vi "Read Configuration.vi"(8 "error in (no error)":errorcluster, 11 "Common Measurements in":refnum<class "Common Measurements.lvclass">) -> (0 "error out":errorcluster, 3 "Common Measurements out":refnum<class "Common Measurements.lvclass">)   [LabVIEW 2015, in "Common Measurements.lvclass"]
uses:
  Common Measurements.lvclass
  <vilib>/Utility/sysdir.llb/System Directory Type.ctl
  Common Measurements.lvclass/Common Measurements.ctl
  <vilib>/Utility/config.llb/Read Key (Boolean).vi
  <vilib>/Utility/config.llb/NI_LVConfig.lvlib
panel:
  out "system directory":path
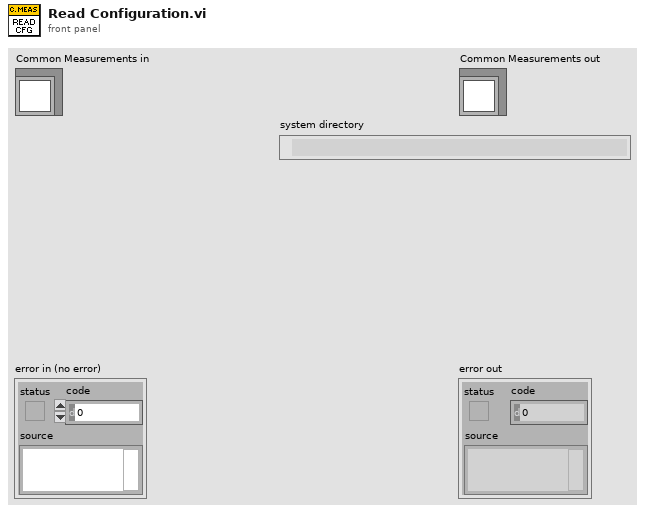
[diagram p1: front panel]
types:
  T1 = typedef "System Directory Type.ctl" = i32
  T2 = typedef "NI_LVConfig.lvlib/Config Data RefNum.ctl" = refnum<k1>
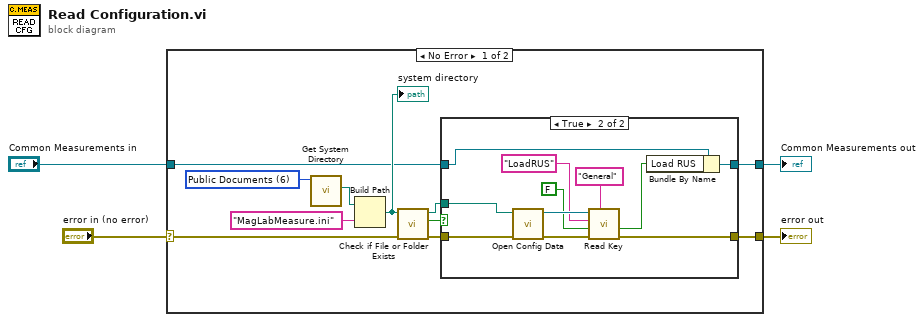
[diagram p0: block diagram]
diagram:
  n1 = case shown="No Error" "error in (no error)" {
    selector: "error in (no error)" -> [w6 w30]
    tunnel: [w5 w30] -> w3
    tunnel: [w8 w29] -> w1
    tunnel: "Common Measurements in" -> [w9 w29]
    frame No Error {
      w15 = T1 6 items=["User Home"=0, "User Desktop"=1, "User Documents"=2, "User Application Data"=3, "User Preferences"=4, "User Temporary"=5, "Public Documents"=6, "Public Application Data"=7, "Public Preferences"=8, "Public Cache"=13, "System Core Libraries"=9, "System Installed Libraries"=10, "Application Files"=11, "Boot Volume Root"=12] ("system directory type")
      n2 = call <vilib>:"Get System Directory.vi"("system directory type"=w15) -> ("system directory"=w14:path)  [unwired: 10 in]
      n3 = Build Path(base path=w14, name or relative path="MagLabMeasure.ini") -> (appended path=w12:path)
      "system directory" <- w12
      n4 = call <vilib>:"Check if File or Folder Exists.vi"("error in (no error)"=w6, "path"=w12) -> ("error out"=w7:errorcluster, "file or folder exists?"=w11:bool, "dup path"=w10:path)  [unwired: 7 in]
      n5 = case shown="True" w11 {
        tunnel: w10 -> [_ w28]
        tunnel: w9 -> [w17 w23]
        tunnel: [w17 w21] -> w8
        tunnel: w7 -> [w16 w20]
        tunnel: [w16 w19] -> w5
        frame False {
        }
        frame True {
          n6 = call <vilib>:"Open Config Data.vi"("error in (no error)"=w20, "configuration file path"=w28) -> ("error out"=w27:errorcluster, "refnum"=w26:T2)  [unwired: 7 in, 1 out]
          n7 = call-poly <vilib>:"Read Key.vi"("section"="General", "error in (no error)"=w27, "default value"=FALSE, "key"="LoadRUS", "refnum"=w26) -> ("error out"=w19:errorcluster, "value"=w22:bool)  [unwired: 3 in, 2 out]
          n8 = Bundle By Name(cluster=w23, "Load RUS"=w22) -> (w21:refnum<class "Common Measurements.lvclass">)
        }
      }
    }
    frame Error {
    }
  }
  "error out" <- w3
  "Common Measurements out" <- w1
